vi "Read StopHelperLoop Reg Ref.vi"(8 "error in (no error)":errorcluster, 11 "Base UI Actor in":refnum<class "Base UI Actor.lvclass">) -> (0 "error out":errorcluster, 2 "StopHelperLoop Reg Ref":refnum<event-registration>, 3 "Base UI Actor out":refnum<class "Base UI Actor.lvclass">)   [LabVIEW 2020, in "Base UI Actor.lvlib" / "Base UI Actor.lvclass"]
uses:
  Base UI Actor.lvclass
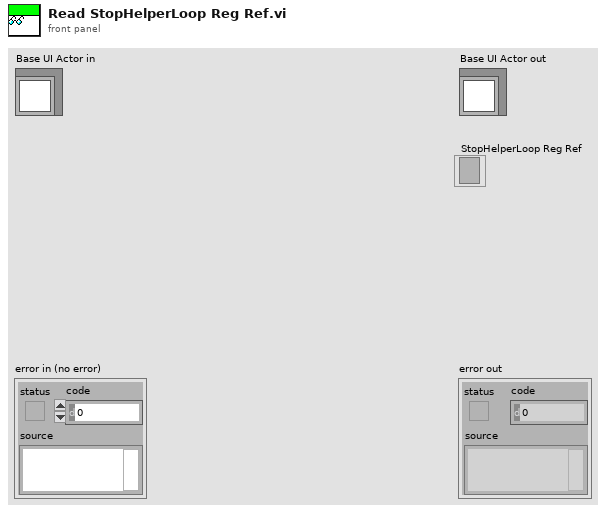
[diagram p1: front panel]
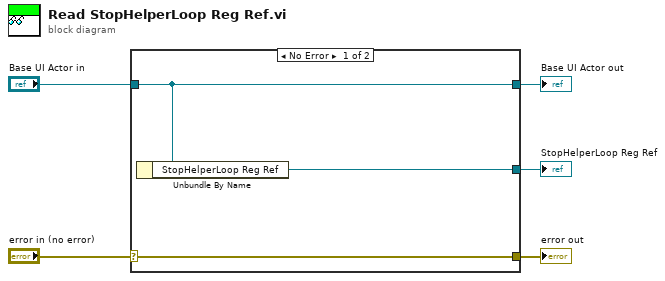
[diagram p0: block diagram]
diagram:
  n1 = case shown="No Error" "error in (no error)" {
    selector: "error in (no error)" -> [w8 w9]
    tunnel: [w8 w9] -> w4
    tunnel: [w7 w10] -> w2
    tunnel: "Base UI Actor in" -> [w7 w10]
    tunnel: [w6 _] -> w1
    frame No Error {
      n2 = Unbundle By Name(w7) -> ("StopHelperLoop Reg Ref"=w6:refnum<event-registration>)
    }
    frame Error {
    }
  }
  "error out" <- w4
  "Base UI Actor out" <- w2
  "StopHelperLoop Reg Ref" <- w1
